vi "GetUseDefaultUI.vi"(8 "error in (no error)":errorcluster, 11 "Device in":refnum<class "Device.lvclass">) -> (0 "error out":errorcluster, 2 "User Default UI?":bool, 3 "Device out":refnum<class "Device.lvclass">)   [LabVIEW 2020, in "Device.lvlib" / "Device.lvclass"]
uses:
  Device.lvclass
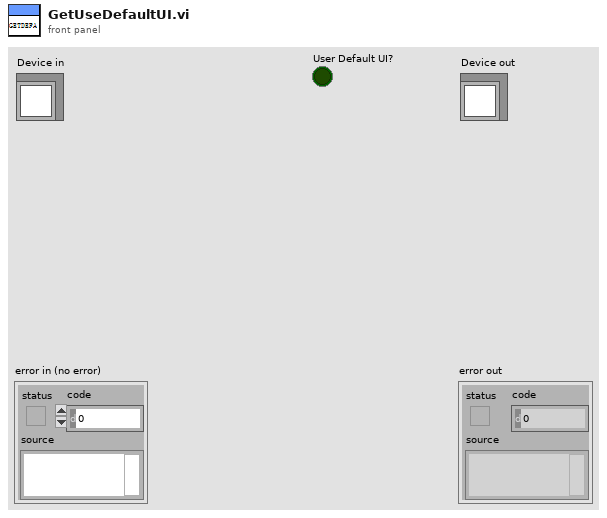
[diagram p1: front panel]
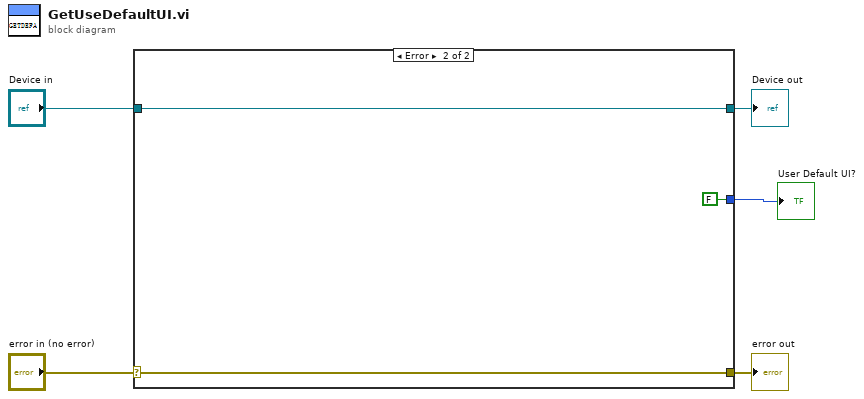
[diagram p0: block diagram]
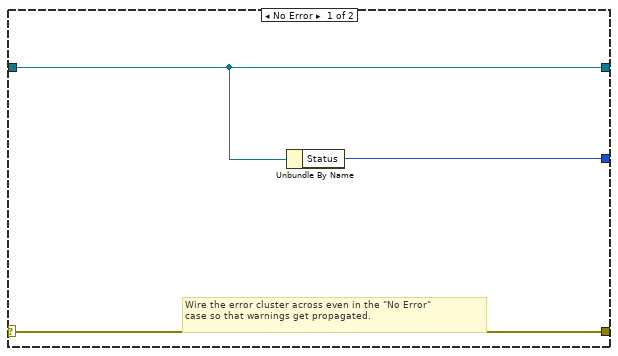
[diagram p2: hidden frame]
diagram:
  n1 = case shown="Error" "error in (no error)" {
    selector: "error in (no error)" -> [w8 w11]
    tunnel: [w8 w11] -> w4
    tunnel: [w7 w10] -> w2
    tunnel: "Device in" -> [w7 w10]
    tunnel: [w6 FALSE ("User Default UI?")] -> w1
    frame No Error {
      # "Wire the error cluster across even in the \"No Error\"\ncase so that warnings get propagated."
      n2 = Unbundle By Name(w7) -> ("Status"=w6:i32)
    }
    frame Error {
    }
  }
  "error out" <- w4
  "Device out" <- w2
  "User Default UI?" <- w1
